vi "SSC Digital Configure HRAM Trigger.vi"(0 "Digital SSC in":T1[](array[typedef]), 5 "Triggers Type":i32(ring)=2200 items=["First Failure"=2200, "Cycle Number"=2201, "Pattern Label"=2202], 7 "Cycle Number Trig:Cycle Number":i64, 9 "Pattern Label Trig:Pattern Label":string, 11 "error in":errorcluster, 12 "Pattern Label Trig:Cycle Offset":i64, 13 "Pattern Label Trig:Vector Offset":i64) -> (4 "Digital SSC out":T1[](array[typedef]), 15 "error out":errorcluster)   [LabVIEW 2019]
doc: "Uses the start label you specify to burst the pattern on the pin(s) and pin group(s) you specify."
uses:
  SSC Digital.ctl
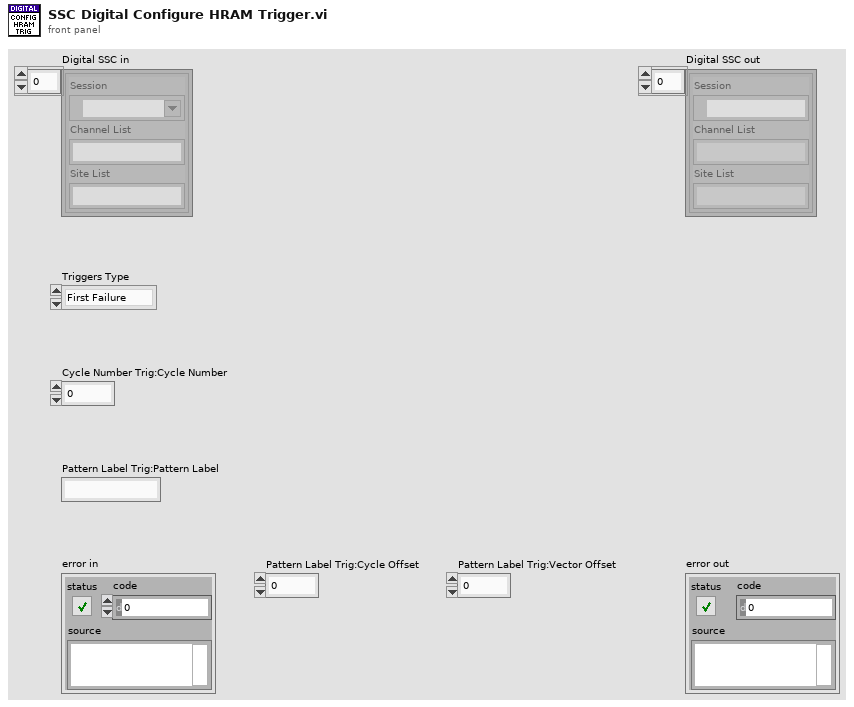
[diagram p1: front panel]
types:
  T1 = typedef "SSC Digital.ctl" = cluster{"Session":refnum<k15>, "Channel List":string, "Site List":string}
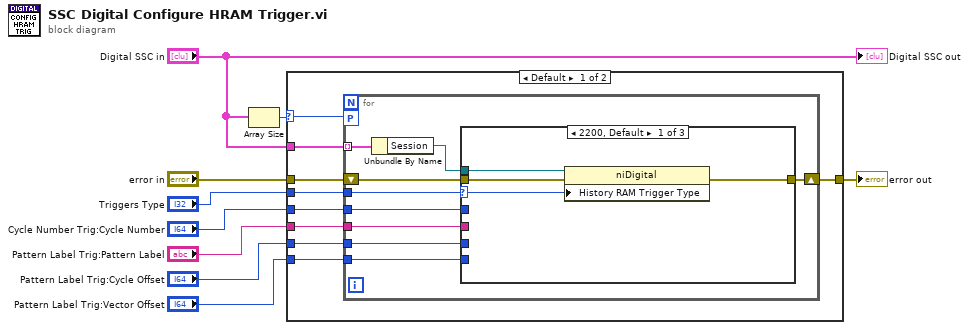
[diagram p0: block diagram]
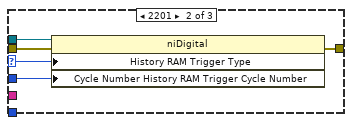
[diagram p2: hidden frame]
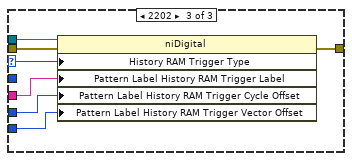
[diagram p3: hidden frame]
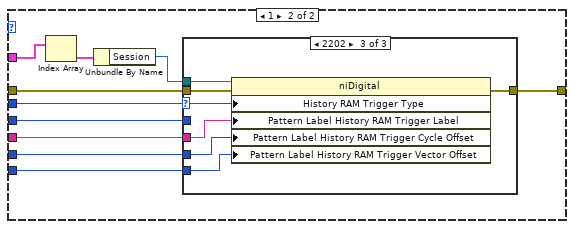
[diagram p4: hidden frame]
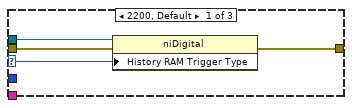
[diagram p5: hidden frame]
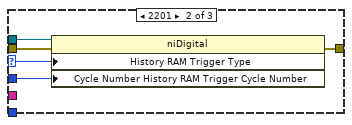
[diagram p6: hidden frame]
diagram:
  n1 = Array Size(array="Digital SSC in") -> (size(s)=w8:i32)
  n2 = case shown="Default" w8 {
    selector: w8 -> [w18 _]
    tunnel: "error in" -> [w16 w52]
    tunnel: "Digital SSC in" -> [w17 w53]
    tunnel: [w15 w51] -> w6
    tunnel: "Triggers Type" -> [w14 w50]
    tunnel: "Cycle Number Trig:Cycle Number" -> [w13 w49]
    tunnel: "Pattern Label Trig:Pattern Label" -> [w12 w48]
    tunnel: "Pattern Label Trig:Cycle Offset" -> [w11 w47]
    tunnel: "Pattern Label Trig:Vector Offset" -> [w10 w46]
    frame Default {
      n3 = for {
        tunnel: w17 -> [w27] mode=indexing
        workers-P: w18 -> [_]
        shift-right: [w26] -> w15
        shift-left: w16 -> [w24]
        tunnel: w14 -> [w23]
        tunnel: w13 -> [w22]
        tunnel: w12 -> [w21]
        tunnel: w11 -> [w20]
        tunnel: w10 -> [w19]
        n4 = Unbundle By Name(w27) -> ("Session"=w25:refnum<k15>)
        n5 = case shown="2200, Default" w23 {
          selector: w23 -> [w28 w33 w40]
          tunnel: [w31 w36 w43] -> w26
          tunnel: w25 -> [w30 w35 w42]
          tunnel: w24 -> [w29 w34 w41]
          tunnel: w22 -> [_ w32 _]
          tunnel: w21 -> [_ _ w39]
          tunnel: w20 -> [_ _ w38]
          tunnel: w19 -> [_ _ w37]
          frame 2200, Default {
            n6 = property class="niDigital"(reference=w30, error in=w29, "History RAM Trigger Type"=w28) -> (error out=w31:errorcluster)  [unwired: 1 out]
          }
          frame 2201 {
            n7 = property class="niDigital"(reference=w35, error in=w34, "History RAM Trigger Type"=w33, "Cycle Number History RAM Trigger Cycle Number"=w32) -> (error out=w36:errorcluster)  [unwired: 1 out]
          }
          frame 2202 {
            n8 = property class="niDigital"(reference=w42, error in=w41, "History RAM Trigger Type"=w40, "Pattern Label History RAM Trigger Label"=w39, "Pattern Label History RAM Trigger Cycle Offset"=w38, "Pattern Label History RAM Trigger Vector Offset"=w37) -> (error out=w43:errorcluster)  [unwired: 1 out]
          }
        }
      }
    }
    frame 1 {
      n9 = Index Array(array=w53) -> (element=w44:T1)  [unwired: 1 in]
      n10 = Unbundle By Name(w44) -> ("Session"=w45:refnum<k15>)
      n11 = case shown="2202" w50 {
        selector: w50 -> [w54 w59 w66]
        tunnel: [w57 w62 w69] -> w51
        tunnel: w45 -> [w56 w61 w68]
        tunnel: w52 -> [w55 w60 w67]
        tunnel: w49 -> [_ w58 _]
        tunnel: w48 -> [_ _ w65]
        tunnel: w47 -> [_ _ w64]
        tunnel: w46 -> [_ _ w63]
        frame 2200, Default {
          n12 = property class="niDigital"(reference=w56, error in=w55, "History RAM Trigger Type"=w54) -> (error out=w57:errorcluster)  [unwired: 1 out]
        }
        frame 2201 {
          n13 = property class="niDigital"(reference=w61, error in=w60, "History RAM Trigger Type"=w59, "Cycle Number History RAM Trigger Cycle Number"=w58) -> (error out=w62:errorcluster)  [unwired: 1 out]
        }
        frame 2202 {
          n14 = property class="niDigital"(reference=w68, error in=w67, "History RAM Trigger Type"=w66, "Pattern Label History RAM Trigger Label"=w65, "Pattern Label History RAM Trigger Cycle Offset"=w64, "Pattern Label History RAM Trigger Vector Offset"=w63) -> (error out=w69:errorcluster)  [unwired: 1 out]
        }
      }
    }
  }
  "error out" <- w6
  "Digital SSC out" <- "Digital SSC in"
